vi "gfitsio-close-file.vi"(8 "error in (no error)":errorcluster, 11 "gfits refnum":T1) -> (0 "error out":errorcluster, 3 "Path":path)   [LabVIEW 2019, in "gfitsio.lvlib"]
doc: "Closes an open file specified by <B>gfits refnum</B>. Error I/O operates uniquely in this function, which closes the file regardless of whether an error occurred in a preceding operation."
uses:
  gfitsio.lvlib
  gfitsio-refnum.ctl
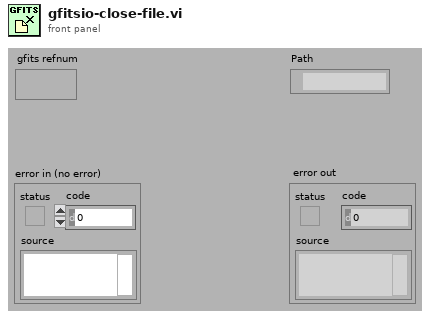
[diagram p1: front panel]
types:
  T1 = typedef "gfitsio.lvlib/gfitsio-refnum.ctl" = refnum<k1>
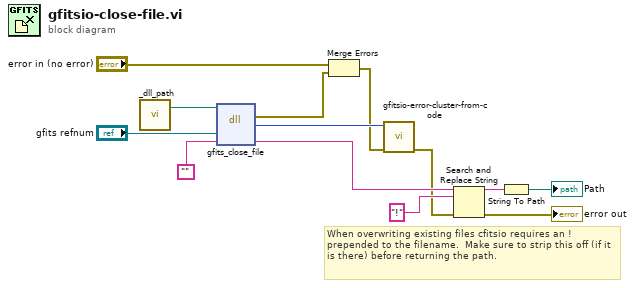
[diagram p0: block diagram]
diagram:
  # "When overwriting existing files cfitsio requires an ! prepended to the filename.  Make sure to strip this off (if it is there) before returning the path."
  n1 = call "_dll_path.vi"() -> ("Path"=w1:path)  [unwired: 1 in]
  n2 = dll-call lib="?" fn="gfits_close_file"(path in=w1, "refnum"="gfits refnum", "path"="") -> (error out=w5:errorcluster, "return type"=w13:i32, "path"=w8:string)  [unwired: 3 in, 1 out]
  n3 = Merge Errors("error in (no error)", w5) -> (w4:errorcluster)
  n4 = call "gfitsio-error-cluster-from-code.vi"("error in (no error)"=w4, "error code"=w13) -> ("error out"=w3:errorcluster)  [unwired: 9 out]
  n5 = Search and Replace String(input string=w8, search string="!", error in=w3) -> (result string=w7:string, error out=→"error out":errorcluster)  [unwired: 5 in, 2 out]
  n6 = String To Path(string=w7) -> (path=→"Path":path)
